vi "TS_FILE_READER_old.VI"(2 "error in (no error)":errorcluster, 3 "File":path) -> (0 "error out":errorcluster, 1 "Data Output":T1={"Comments"="", "Ref Impedance"=75, "Trace Array"=[]} {"Trace Array"."Freq (Hz)" format="%.2e"; "Trace Array"."S-parameter Array" format="%.2f"})   [LabVIEW 2017]
doc: "Writes data in Freq S Real Imag or Magnitude Angle \n9 Column Touchstone format \nfeatures write protection for existing files"
panel:
  out "Data Format":enum16{"RI", "MA", "dB"}(ring)
  out "Freq Multiplier":dbl
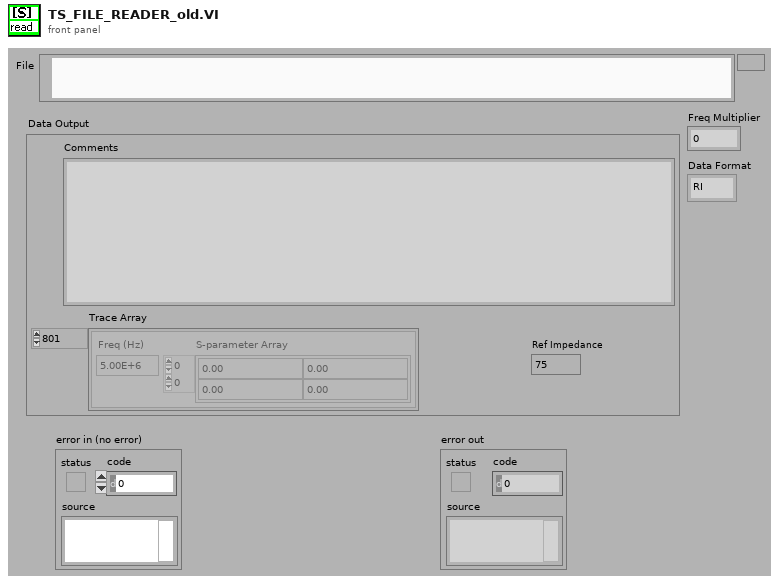
[diagram p1: front panel]
types:
  T1 = cluster{"Comments":string, "Ref Impedance":u16, "Trace Array":cluster{"Freq (Hz)":dbl, "S-parameter Array":cdb[][]}[]}
  T2 = cluster{"Freq (Hz)":dbl, "S-parameter Array":cdb[][]}[]
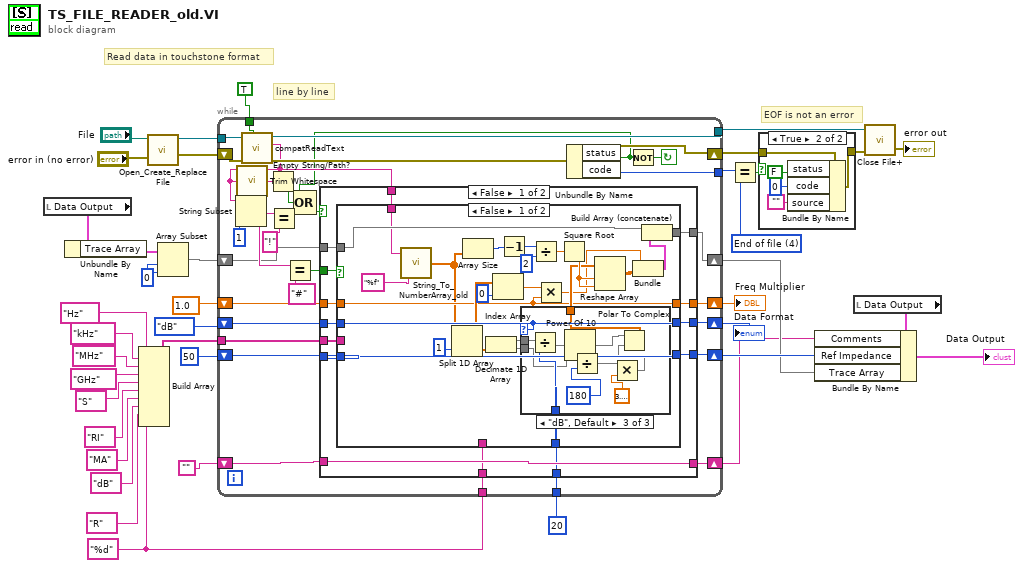
[diagram p0: block diagram]
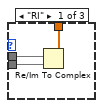
[diagram p3: hidden frame]
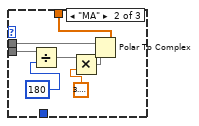
[diagram p4: hidden frame]
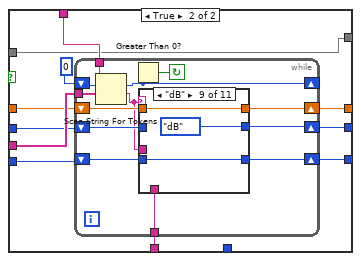
[diagram p5: hidden frame]
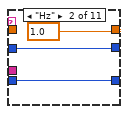
[diagram p7: hidden frame]
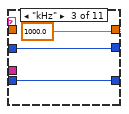
[diagram p8: hidden frame]
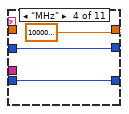
[diagram p9: hidden frame]
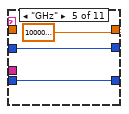
[diagram p10: hidden frame]
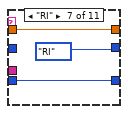
[diagram p12: hidden frame]
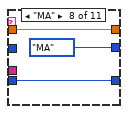
[diagram p13: hidden frame]
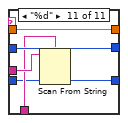
[diagram p15: hidden frame]
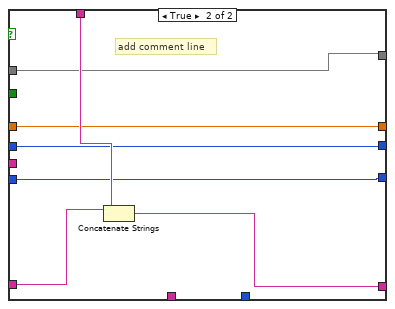
[diagram p16: hidden frame]
diagram:
  w10 = 0
  w17 = "%d"
  w32 = 4 items=["No error", "Argument error", "Memory is full", "Out of zone", "End of file", "File already open", "Generic file I/O error", "File not found", "File permission error", "Disk is full", "Duplicate path", "Too many files open", "System feature not enabled", "Resource file not found", "Cannot add resource", "Resource not found", "Image not found", "Image memory error", "Pen does not exist", "Config type invalid", "Config token not found", "Config parse error", "Config memory error", "Bad external code format", "Bad external code offset", "External code not present", "Null window", "Destroy window error", "Null menu", "Print aborted", "Bad print record", "Print driver error", "Windows error during printing", "Memory error during printing", "Print dialog error", "Generic print error", "Invalid device refnum", "Device not found", "Device parameter error", "Device unit error", "Cannot open device", "Device call aborted", "Generic error", "Cancelled by user", "Object ID too low", "Object ID too high", "Object not in heap", "Unknown heap", "Unknown object (invalid DefProc)", "Unknown object (DefProc not in table)", "Message out of range", "Invalid (null) method", "Unknown message", "Manager call not supported", "Bad address", "Network operation in progress", "Network operation timed out", "Connection is busy", "Network attribute not supported", "Network error", "Address in use", "System out of memory", "Connection aborted", "Connection refused", "Not connected", "Already connected", "Connection closed", "Initialization error (interapplication manager)", "Bad occurrence", "Wait on unbound occurrence handler", "Occurrence queue overflow", "Datalog type conflict", "Unused", "Unrecognized type (interapplication manager)", "Memory corrupt", "Failed to make temporary DLL", "Old CIN version", "Drag socket not found", "Failed to load drop-object", "Failed to register OLE object", "Failed to release OLE object", "Format specifier type mismatch", "Unknown format specifier", "Too few format specifiers", "Too many format specifiers", "Scan failed", "Newer CIN version", "Error converting to variant", "Runtime menu error", "Password tampered", "Variant attribute not found", "Incompatible variant data type", "Event data is not available", "Event Store is not present", "Occurrence is not found", "Event Queue is not created", "Event info is not available", "Refnum passed is NULL", "Error retrieving Class GUID", "Error retrieving CoClass GUID", "Error retrieving TypeLib GUID.", "Bad built application magic bytes.", "Specific driver is different from the specific driver associated with the Logical Name.", "There is no session opened to the class driver.", "Max Error", "MAX - Error with config objects", "MAX - Error loading configuration", "MAX - Group not supported"]
  # "line by line"
  # "EOF is not an error"
  # "Read data in touchstone format"
  n1 = local read "Data Output"() -> (w13:T1)
  n2 = Unbundle By Name(w13) -> ("Trace Array"=w12:T2)
  n3 = Build Array("Hz", "kHz", "MHz", "GHz", "S", "RI", "MA", "dB", "R", w17) -> (w18:string[])
  n4 = call <vilib>:"Open_Create_Replace File.vi"("error in (no error)"="error in (no error)", "file path"="File") -> ("error out"=w36:errorcluster, "refnum"=w38:refnum<file>)  [unwired: 4 in, 4 out]
  n5 = Array Subset(array=w12, index=w10, length=w10) -> (w11:T2)
  n6 = while {
    tunnel: [w68] -> w30
    tunnel: w38 -> [w70]
    tunnel: TRUE -> [w69]
    shift-right: [w66] -> w29
    shift-left: w36 -> [w67]
    tunnel: [w64] -> w33
    tunnel: w18 -> [w58]
    tunnel: w17 -> [w57]
    shift-right: [w54] -> w2
    shift-left: 1.0 -> [w55]
    shift-right: [w53] -> w14
    shift-left: u16 50 -> [w56]
    shift-right: [w51] -> w1
    shift-left: enum16{"RI", "MA", "dB"}."dB" -> [w52]
    shift-right: [w49] -> w9
    shift-left: w11 -> [w50]
    shift-right: [w47] -> w7
    shift-left: "" -> [w48]
    tunnel: 20 -> [w46]
    stop <- w65 continue-if-true
    n7 = call <vilib>:"compatReadText.vi"("line mode (F)"=w69, "error in"=w67, "refnum"=w70) -> ("error out"=w66:errorcluster, "data"=w44:string, "dup refnum"=w68:refnum<file>)  [unwired: 2 in, 4 out]
    n8 = String Subset(string=w44, length (rest)=1) -> (substring=w62:string)  [unwired: 1 out]
    n9 = call <vilib>:"Trim Whitespace.vi"("string"=w44) -> ("trimmed string"=w45:string)  [unwired: 1 in]
    n10 = Empty String/Path?(string/path=w45) -> (empty?=w41:bool)
    n11 = Equal?(x=w62, y="!") -> (x = y?=w40:bool)
    n12 = Equal?(x=w62, y="#") -> (x = y?=w60:bool)
    n13 = Unbundle By Name(w66) -> ("status"=w42:bool, "code"=w64:i32)
    n14 = Compound Arithmetic op=OR(w42, w41, w40) -> (w43:bool)
    n15 = case shown="False" w43 {
      tunnel: w48 -> [w84 w195]
      tunnel: [w84 w194] -> w47
      tunnel: w44 -> [w82 w196]
      tunnel: w60 -> [w83 _]
      tunnel: w58 -> [w81 _]
      tunnel: w57 -> [w80 _]
      tunnel: [w79 w193] -> w53
      tunnel: w56 -> [w78 w193]
      tunnel: w55 -> [w77 w192]
      tunnel: [w76 w192] -> w54
      tunnel: w52 -> [w75 w191]
      tunnel: [w74 w191] -> w51
      tunnel: w50 -> [w73 w190]
      tunnel: [w72 w190] -> w49
      tunnel: w46 -> [w71 _]
      frame False {
        n16 = case shown="False" w83 {
          tunnel: w82 -> [w87 w140]
          tunnel: w81 -> [_ w139]
          tunnel: w80 -> [_ w138]
          tunnel: [w109 w137] -> w79
          tunnel: w78 -> [w109 w136]
          tunnel: w77 -> [w89 w135]
          tunnel: [w89 w134] -> w76
          tunnel: w75 -> [w101 w132]
          tunnel: [w101 w131] -> w74
          tunnel: w73 -> [w97 w130]
          tunnel: [w92 w130] -> w72
          tunnel: w71 -> [w88 _]
          frame False {
            n17 = call "String_To_NumberArray_old.vi"("Format"="%f", "Input String"=w87) -> ("Output Array"=w86:dbl[])
            n18 = Split 1D Array(array=w86, index=1) -> (first subarray=w94:dbl[], second subarray=w102:dbl[])
            n19 = Array Size(array=w86) -> (size(s)=w108:i32)
            n20 = Decimate 1D Array(w102) -> (w100:dbl[], w99:dbl[])
            n21 = Index Array(array=w94, index=0) -> (element=w90:dbl)
            n22 = Decrement(x=w108) -> (x-1=w107:i32)
            n23 = case shown="\"dB\", Default" w101 {
              tunnel: w100 -> [w112 w119 w128]
              tunnel: w99 -> [w111 w117 w121]
              tunnel: [w110 w118 w129] -> w98
              tunnel: w88 -> [_ _ w127]
              frame "RI" {
                n24 = Re/Im To Complex(1:w111, 2:w112) -> (0:w110:cdb[])
              }
              frame "MA" {
                n25 = Divide(x=w117, y=180) -> (x/y=w115:dbl[])
                n26 = Multiply(x=w115, y=3.141592653589793) -> (x*y=w113:dbl[])
                n27 = Polar To Complex(1:w113, 2:w119) -> (0:w118:cdb[])
              }
              frame "dB", Default {
                n28 = Divide(x=w128, y=w127) -> (x/y=w126:dbl[])
                n29 = Power Of 10(x=w126) -> (10^x=w125:dbl[])
                n30 = Divide(x=w121, y=180) -> (x/y=w123:dbl[])
                n31 = Multiply(x=w123, y=3.141592653589793) -> (x*y=w120:dbl[])
                n32 = Polar To Complex(1:w120, 2:w125) -> (0:w129:cdb[])
              }
            }
            n33 = Divide(x=w107, y=2) -> (x/y=w105:dbl)
            n34 = Multiply(x=w90, y=w89) -> (x*y=w91:dbl)
            n35 = Square Root(x=w105) -> (sqrt(x)=w103:dbl)
            n36 = Reshape Array(w98, w103, w103) -> (w96:cdb[][])
            n37 = Bundle(w91, w96) -> (w95:cluster{dbl, cdb[][]})  [unwired: 1 out]
            n38 = Build Array (concatenate)(w97, w95) -> (w92:T2)
          }
          frame True {
            n39 = while {
              shift-right: [w150] -> _
              shift-left: 0 -> [w152]
              tunnel: w140 -> [w153]
              tunnel: w139 -> [w149]
              shift-right: [w148] -> w134
              shift-left: w135 -> [w147]
              shift-right: [w146] -> w131
              shift-left: w132 -> [w145]
              tunnel: w138 -> [w144]
              shift-right: [w143] -> w137
              shift-left: w136 -> [w142]
              stop <- w151 continue-if-true
              n40 = Scan String For Tokens(7:w149, 8:w152, 9:w153) -> (1:w141:string, 2:w150:i32)  [unwired: 5 out]
              n41 = Greater Than 0?(x=w150) -> (x > 0?=w151:bool)
              n42 = case shown="\"dB\"" w141 {
                tunnel: [w156 1.0 1000.0 1000000.0 1000000000.0 w171 w174 w177 w180 w183 w189] -> w148
                tunnel: w147 -> [w156 _ _ _ _ w171 w174 w177 w180 w183 w189]
                tunnel: [w155 w158 w161 w164 w167 w170 enum16{"RI", "MA", "dB"}."RI" enum16{"RI", "MA", "dB"}."MA" enum16{"RI", "MA", "dB"}."dB" w182 w188] -> w146
                tunnel: w145 -> [w155 w158 w161 w164 w167 w170 _ _ _ w182 w188]
                tunnel: w141 -> [_ _ _ _ _ _ _ _ _ _ w187]
                tunnel: w144 -> [_ _ _ _ _ _ _ _ _ _ w186]
                tunnel: [w154 w157 w160 w163 w166 w169 w173 w176 w179 w181 w185] -> w143
                tunnel: w142 -> [w154 w157 w160 w163 w166 w169 w173 w176 w179 w181 w184]
                frame Default {
                }
                frame "Hz" {
                }
                frame "kHz" {
                }
                frame "MHz" {
                }
                frame "GHz" {
                }
                frame "S" {
                }
                frame "RI" {
                }
                frame "MA" {
                }
                frame "dB" {
                }
                frame "R" {
                }
                frame "%d" {
                  n43 = Scan From String(format string=w186, input string=w187, default 1=w184) -> (output 1=w185:u16)  [unwired: 2 in, 3 out]
                }
              }
            }
          }
        }
      }
      frame True {
        # "add comment line"
        n44 = Concatenate Strings(w195, w196) -> (w194:string)
      }
    }
    n45 = Not(x=w42) -> (.not. x?=w65:bool)
  }
  "Freq Multiplier" <- w2
  "Data Format" <- w1
  n46 = Equal?(x=w33, y=w32) -> (x = y?=w31:bool)
  n47 = case shown="True" w31 {
    tunnel: w29 -> [w197 w202]
    tunnel: [w197 w198] -> w28
    frame False {
    }
    frame True {
      n48 = Bundle By Name(cluster=w202, "status"=FALSE, "code"=0, "source"="") -> (w198:errorcluster)
    }
  }
  n49 = local read "Data Output"() -> (w26:T1)
  n50 = Bundle By Name(cluster=w26, "Comments"=w7, "Ref Impedance"=w14, "Trace Array"=w9) -> (→"Data Output":T1)
  n51 = call <vilib>:"Close File+.vi"("error in (no error)"=w28, "refnum"=w30) -> ("error out"=→"error out":errorcluster)  [unwired: 5 out]
